vi "Handle Last Ack Core.vi"(4 "error in (no error)":errorcluster, 6 "Last Ack":refnum<class "Last Ack.lvclass">, 7 "Actor in":refnum<class "Actor.lvclass">) -> (0 "error out":errorcluster, 3 "Actor out":refnum<class "Actor.lvclass">)   [LabVIEW 2020, in "Actor Framework.lvlib" / "Actor.lvclass"]
doc: "<p>(<strong>Filename</strong>: <span class=\"dnl\">Actor Framework.lvlib:Actor.lvclass:Handle Last Ack Core.vi</span>)</p>\n<p>Defines how the caller actor responds to the Last Ack message from a nested actor. The Last Ack message is the final message a nested actor sends to its caller before it shuts down. The message contains information about the final state of the nested actor.</p>\n<p>By default, this method does nothing except return any error the nested actor sent. A descendant class may override this method to define behavior.</p>"
uses:
  Actor.lvclass
  LastAck/Last Ack.lvclass
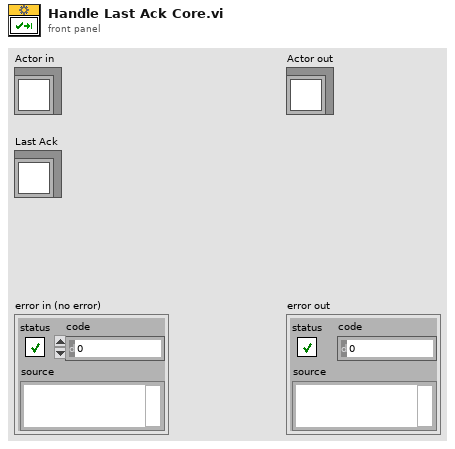
[diagram p1: front panel]
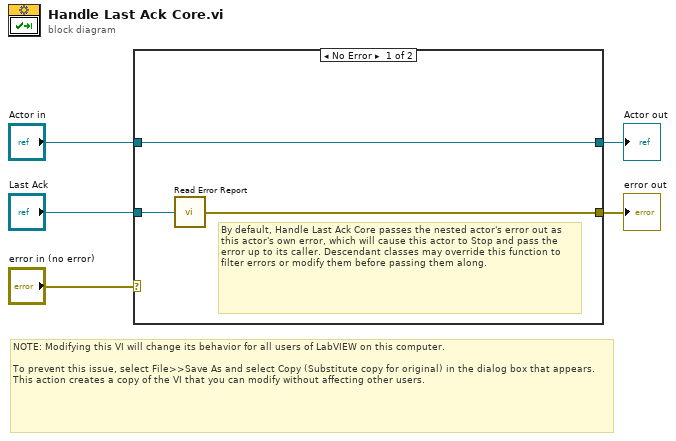
[diagram p0: block diagram]
diagram:
  # "NOTE: Modifying this VI will change its behavior for all users of LabVIEW on this computer.\n\nTo prevent this issue, select File>>Save As and select Copy (Substitute copy for original) in the dialog box that appears. This action creates a copy of the VI that you can modify without affecting other users."
  n1 = case shown="No Error" "error in (no error)" {
    selector: "error in (no error)" -> [_ w10]
    tunnel: [w7 w10] -> w2
    tunnel: [w6 w9] -> w4
    tunnel: "Actor in" -> [w6 w9]
    tunnel: "Last Ack" -> [w8 _]
    frame No Error {
      # "By default, Handle Last Ack Core passes the nested actor's error out as this actor's own error, which will cause this actor to Stop and pass the error up to its caller. Descendant classes may override this function to filter errors or modify them before passing them along."
      n2 = call "Read Error Report.vi"("Last Ack"=w8) -> ("error report"=w7:errorcluster)
    }
    frame Error {
    }
  }
  "Actor out" <- w4
  "error out" <- w2
